vi "onConnection.vi"(8 "error in (no error)":errorcluster, 11 "WSConnection in":refnum<class "WebsocketsConnection.lvclass">) -> (0 "error out":errorcluster, 3 "WSConnection":refnum<class "WebsocketsConnection.lvclass">)   [LabVIEW 2013, in "MQTT_Websockets.lvlib" / "WebsocketsConnection.lvclass"]
uses:
  WebsocketsConnection.lvclass
  MQTT_Connection/Connection/Connection.lvclass
  WebsocketsConnection.lvclass/WebsocketsConnection.ctl
  <vilib>/MediaMongrels Ltd/WebSockets/WebSockets/WebSocket/WebSocket.lvclass/WebSocket.ctl
  MQTT_Connection/Connection/Connection.lvclass/Connection.ctl
  <vilib>/MediaMongrels Ltd/WebSockets/WebSockets/WebSocket Client/WebSocket Client.lvclass
  <vilib>/MediaMongrels Ltd/WebSockets/WebSockets/WebSocket/Read Return Headers.vi
  <vilib>/MediaMongrels Ltd/WebSockets/Sockets/VISA TCP Socket/VISA TCP.lvclass
  <vilib>/MediaMongrels Ltd/WebSockets/WebSockets/WebSocket/WebSocket.lvclass
panel:
  out "Return Headers":variant
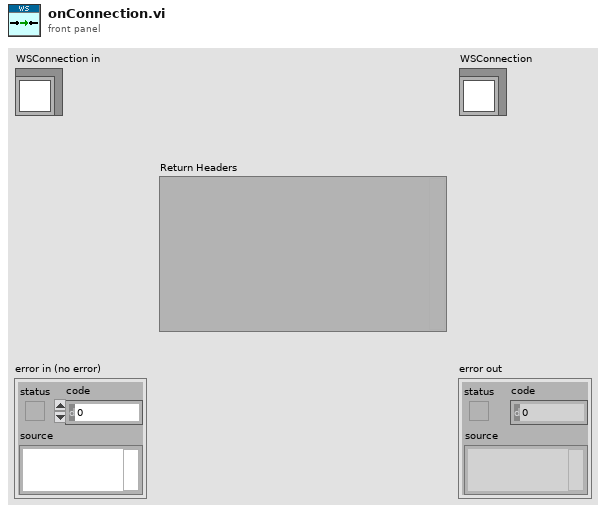
[diagram p1: front panel]
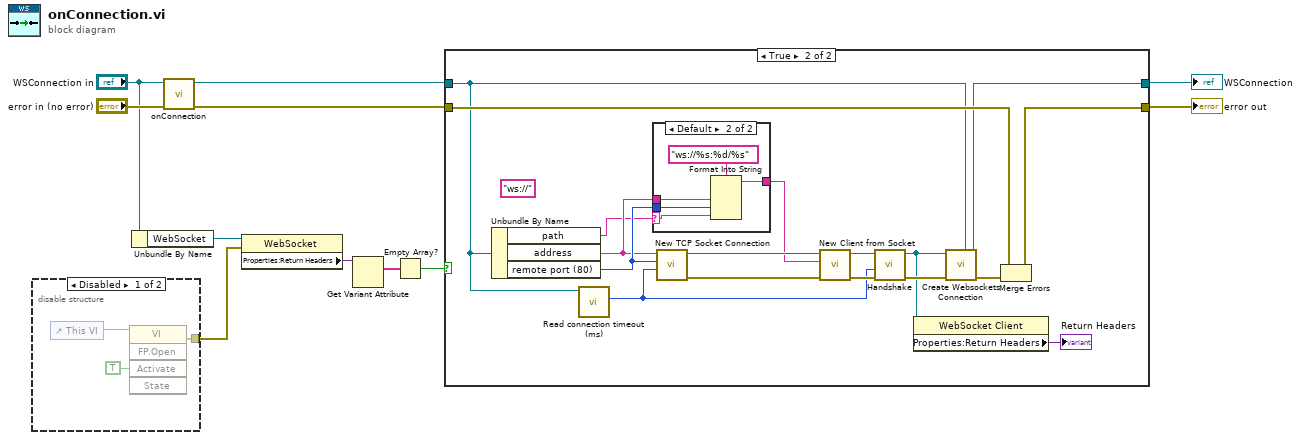
[diagram p0: block diagram]
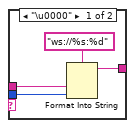
[diagram p4: hidden frame]
diagram:
  n1 = disable-structure shown="Disabled" {
    disable-tunnel: [w12 _] -> w1
    frame Disabled {
      n2 = control-ref of="This VI"() -> (w14:refnum<vi>)
      n3 = invoke class="VI" method="FP.Open"(reference=w14, "Activate"=TRUE ("Activate?")) -> (error out=w12:errorcluster)  [unwired: 3 in, 4 out]
    }
    frame Enabled {
    }
  }
  n4 = Unbundle By Name("WSConnection in") -> ("WebSocket"=w5:refnum<class "WebSocket.lvclass">)
  n5 = call-parent "onConnection.vi"("error in (no error)"="error in (no error)", "Connection in"="WSConnection in") -> ("error out"=w10:errorcluster, "Connection out"=w8:refnum<class "WebsocketsConnection.lvclass">)  [unwired: 8 in]
  n6 = property class="WebSocket"(reference=w5, error in=w1) -> ("Properties:Return Headers"=w4:variant)  [unwired: 2 out]
  n7 = Get Variant Attribute(Variant=w4) -> (names=w3:string[])  [unwired: 3 in, 3 out]
  n8 = Empty Array?(array=w3) -> (empty?=w2:bool)
  n9 = case shown="True" w2 {
    tunnel: w10 -> [w15 w32]
    tunnel: [w15 w30] -> w9
    tunnel: w8 -> [w16 w31]
    tunnel: [w16 w29] -> w7
    frame False {
    }
    frame True {
      (unwired) "ws://" ("string")
      n10 = Unbundle By Name(w31) -> ("path"=w17:string, "address"=w18:string, "remote port (80)"=w20:u16)
      n11 = call "Read connection timeout (ms).vi"("Connection in"=w31) -> ("connection timeout (ms)"=w21:i32)  [unwired: 8 in, 2 out]
      n12 = case shown="Default" w17 {
        selector: w17 -> [_ w38]
        tunnel: w20 -> [w37 w42]
        tunnel: [w36 w41] -> w19
        tunnel: w18 -> [w34 w39]
        frame "\u0000" {
          n13 = Format Into String(format string="ws://%s:%d", w34, w37) -> (resulting string=w36:string)  [unwired: 2 in, 1 out]
        }
        frame Default {
          n14 = Format Into String(format string="ws://%s:%d/%s", w39, w42, w38) -> (resulting string=w41:string)  [unwired: 2 in, 1 out]
        }
      }
      n15 = call <vilib>:"New TCP Socket Connection.vi"("timeout ms (5000)"=w21, "Port"=w20, "Hostname / IP"=w18) -> ("error out"=w27:errorcluster, "VISA TCP out"=w28:refnum<class "VISA TCP.lvclass">)  [unwired: 7 in]
      n16 = call <vilib>:"New Client from Socket.vi"("error in (no error)"=w27, "WebSocket URL"=w19, "Socket in"=w28) -> ("error out"=w26:errorcluster, "WebSocket Client out"=w24:refnum<class "WebSocket Client.lvclass">)  [unwired: 7 in]
      n17 = call-dynamic "Handshake.vi"("error in (no error)"=w26, "timeout ms (5000)"=w21, "WebSocket Client in"=w24) -> ("error out"=w25:errorcluster, "WebSocket Client out"=w23:refnum<class "WebSocket Client.lvclass">)  [unwired: 7 in]
      n18 = property class="WebSocket Client"(reference=w23) -> ("Properties:Return Headers"=→"Return Headers":variant)  [unwired: 1 in, 2 out]
      n19 = call "Create Websockets Connection.vi"("WSConnection in"=w31, "error in (no error)"=w25, "WebSocket"=w23) -> ("error out"=w33:errorcluster, "WSConnection"=w29:refnum<class "WebsocketsConnection.lvclass">)  [unwired: 7 in]
      n20 = Merge Errors(w32, w33) -> (w30:errorcluster)
    }
  }
  "error out" <- w9
  "WSConnection" <- w7
